vi "Get Device Info.vi"(8 "error in (no error)":errorcluster) -> (0 "error out":errorcluster, 2 "Success":bool, 3 "device info":T2 {"in_ver" format="%.2f"; "dr_ver" format="%.2f"; "fw_ver" format="%.2f"; "hw_ver" format="%.2f"})   [LabVIEW 2018, in "CAN FD.lvlib"]
uses:
  CAN FD.lvlib
  data_type/ZCAN_DEVICE_INFO.ctl
  bin/ControlCANFD.dll
panel:
  in  "ZCAN_DEVICE_INFO":T1
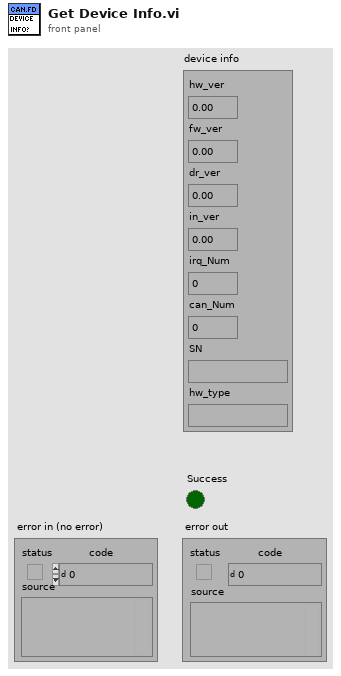
[diagram p1: front panel]
types:
  T1 = typedef "ZCAN_DEVICE_INFO.ctl" = cluster{"hw_Version":u16, "fw_Version":u16, "dr_Version":u16, "in_Version":u16, "irq_Num":u16, "can_Num":u8, "str_Serial_Num":cluster{"str_Serial_Num[0]":u8, "str_Serial_Num[1]":u8, "str_Serial_Num[2]":u8, "str_Serial_Num[3]":u8, "str_Serial_Num[4]":u8, "str_Serial_Num[5]":u8, "str_Serial_Num[6]":u8, "str_Serial_Num[7]":u8, "str_Serial_Num[8]":u8, "str_Serial_Num[9]":u8, "str_Serial_Num[10]":u8, "str_Serial_Num[11]":u8, "str_Serial_Num[12]":u8, "str_Serial_Num[13]":u8, "str_Serial_Num[14]":u8, "str_Serial_Num[15] ":u8, "str_Serial_Num[16] ":u8, "str_Serial_Num[17] ":u8, "str_Serial_Num[18] ":u8, "str_Serial_Num[19]":u8}, "str_hw_Type":cluster{"str_hw_Type[0]":u8, "str_hw_Type[1]":u8, "str_hw_Type[2]":u8, "str_hw_Type[3]":u8, "str_hw_Type[4]":u8, "str_hw_Type[5]":u8, "str_hw_Type[6]":u8, "str_hw_Type[7]":u8, "str_hw_Type[8]":u8, "str_hw_Type[9]":u8, "str_hw_Type[10]":u8, "str_hw_Type[11]":u8, "str_hw_Type[12]":u8, "str_hw_Type[13]":u8, "str_hw_Type[14]":u8, "str_hw_Type[15] ":u8, "str_hw_Type[16] ":u8, "str_hw_Type[17] ":u8, "str_hw_Type[18] ":u8, "str_hw_Type[19]":u8, "str_hw_Type[20]":u8, "str_hw_Type[21]":u8, "str_hw_Type[22]":u8, "str_hw_Type[23]":u8, "str_hw_Type[24]":u8, "str_hw_Type[25]":u8, "str_hw_Type[26]":u8, "str_hw_Type[27]":u8, "str_hw_Type[28]":u8, "str_hw_Type[29]":u8, "str_hw_Type[30]":u8, "str_hw_Type[31]":u8, "str_hw_Type[32]":u8, "str_hw_Type[33]":u8, "str_hw_Type[34]":u8, "str_hw_Type[35] ":u8, "str_hw_Type[36] ":u8, "str_hw_Type[37] ":u8, "str_hw_Type[38] ":u8, "str_hw_Type[39]":u8}, "reserved":cluster{"reserved[0]":u16, "reserved[1] ":u16, "reserved[2] ":u16, "reserved[3] ":u16}}
  T2 = cluster{"hw_ver":dbl, "fw_ver":dbl, "dr_ver":dbl, "in_ver":dbl, "irq_Num":u16, "can_Num":u8, "SN":string, "hw_type":string}
  T3 = cluster{"str_Serial_Num[0]":u8, "str_Serial_Num[1]":u8, "str_Serial_Num[2]":u8, "str_Serial_Num[3]":u8, "str_Serial_Num[4]":u8, "str_Serial_Num[5]":u8, "str_Serial_Num[6]":u8, "str_Serial_Num[7]":u8, "str_Serial_Num[8]":u8, "str_Serial_Num[9]":u8, "str_Serial_Num[10]":u8, "str_Serial_Num[11]":u8, "str_Serial_Num[12]":u8, "str_Serial_Num[13]":u8, "str_Serial_Num[14]":u8, "str_Serial_Num[15] ":u8, "str_Serial_Num[16] ":u8, "str_Serial_Num[17] ":u8, "str_Serial_Num[18] ":u8, "str_Serial_Num[19]":u8}
  T4 = cluster{"str_hw_Type[0]":u8, "str_hw_Type[1]":u8, "str_hw_Type[2]":u8, "str_hw_Type[3]":u8, "str_hw_Type[4]":u8, "str_hw_Type[5]":u8, "str_hw_Type[6]":u8, "str_hw_Type[7]":u8, "str_hw_Type[8]":u8, "str_hw_Type[9]":u8, "str_hw_Type[10]":u8, "str_hw_Type[11]":u8, "str_hw_Type[12]":u8, "str_hw_Type[13]":u8, "str_hw_Type[14]":u8, "str_hw_Type[15] ":u8, "str_hw_Type[16] ":u8, "str_hw_Type[17] ":u8, "str_hw_Type[18] ":u8, "str_hw_Type[19]":u8, "str_hw_Type[20]":u8, "str_hw_Type[21]":u8, "str_hw_Type[22]":u8, "str_hw_Type[23]":u8, "str_hw_Type[24]":u8, "str_hw_Type[25]":u8, "str_hw_Type[26]":u8, "str_hw_Type[27]":u8, "str_hw_Type[28]":u8, "str_hw_Type[29]":u8, "str_hw_Type[30]":u8, "str_hw_Type[31]":u8, "str_hw_Type[32]":u8, "str_hw_Type[33]":u8, "str_hw_Type[34]":u8, "str_hw_Type[35] ":u8, "str_hw_Type[36] ":u8, "str_hw_Type[37] ":u8, "str_hw_Type[38] ":u8, "str_hw_Type[39]":u8}
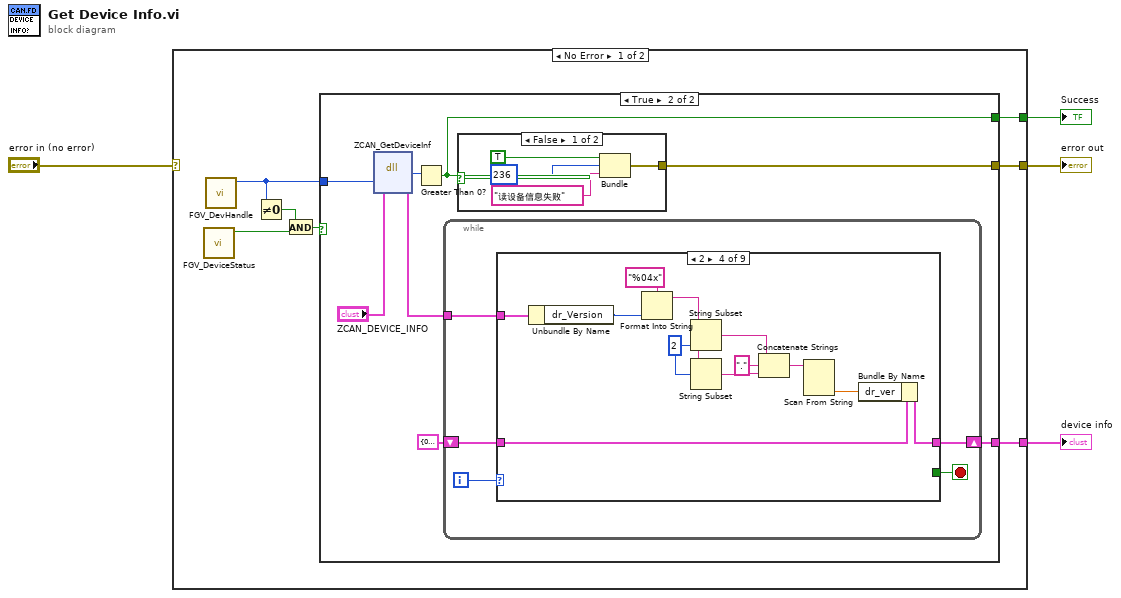
[diagram p0: block diagram]
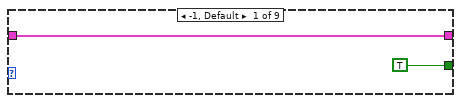
[diagram p3: hidden frame]
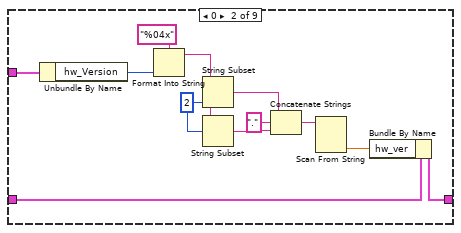
[diagram p4: hidden frame]
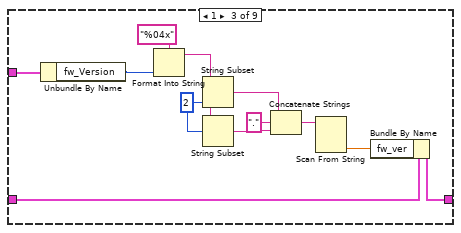
[diagram p5: hidden frame]
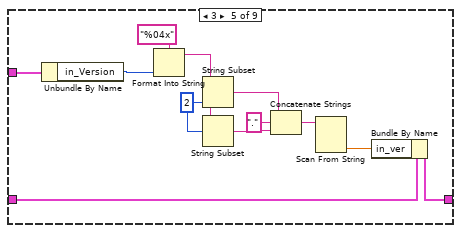
[diagram p6: hidden frame]
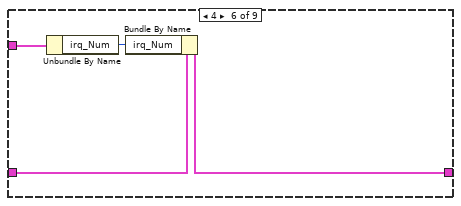
[diagram p7: hidden frame]
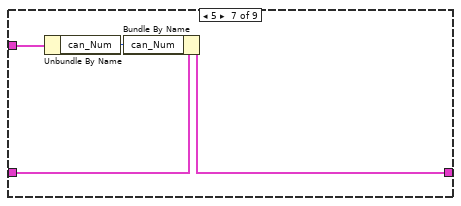
[diagram p8: hidden frame]
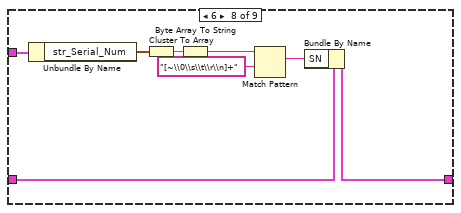
[diagram p9: hidden frame]
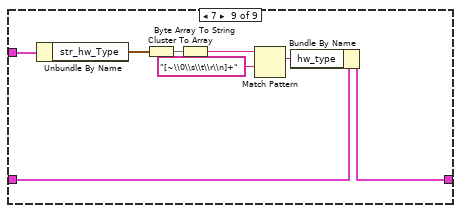
[diagram p10: hidden frame]
diagram:
  n1 = case shown="No Error" "error in (no error)" {
    selector: "error in (no error)" -> [_ w103]
    tunnel: [w8 w103] -> w4
    tunnel: [w7 _] -> w3
    tunnel: [w6 _] -> w2
    frame No Error {
      n2 = call "FGV_DeviceStatus.vi"() -> ("Open?"=w11:bool)  [unwired: 10 in, 1 out]
      n3 = call "FGV_DevHandle.vi"() -> ("handle out"=w9:u64)  [unwired: 9 in, 2 out]
      n4 = Not Equal To 0?(x=w9) -> (x != 0?=w10:bool)
      n5 = And(x=w10, y=w11) -> (x .and. y?=w5:bool)
      n6 = case shown="True" w5 {
        tunnel: w9 -> [_ w12]
        tunnel: [_ w17] -> w8
        tunnel: [_ w16] -> w7
        tunnel: [_ w14] -> w6
        frame False {
        }
        frame True {
          n7 = dll-call lib="C:/Users/ttc52/Desktop/DHC FD LV2018/LABIVIEW CANFD Tool_V1.2.4_20220724/bin/ControlCANFD.dll" fn="ZCAN_GetDeviceInf"("channel_handle"=w12, "pInfo"="ZCAN_DEVICE_INFO") -> ("return"=w19:u32, "pInfo"=w13:T1)  [unwired: 4 in, 2 out]
          n8 = Greater Than 0?(x=w19) -> (x > 0?=w16:bool)
          n9 = while {
            shift-right: [w23] -> w14
            shift-left: T2 {"hw_ver"=0.0, "fw_ver"=0.0, "dr_ver"=0.0, "in_ver"=0.0, "irq_Num"=0, "can_Num"=0, "SN"="", "hw_type"=""} ("device info") -> [w22]
            tunnel: w13 -> [w20]
            i -> [w24]
            stop <- w21 stop-if-true
            n10 = case shown="2" w24 {
              tunnel: [w26 w27 w39 w51 w63 w76 w80 w88 w96] -> w23
              tunnel: w22 -> [w26 w29 w41 w53 w65 w77 w81 w89 w97]
              tunnel: [TRUE _ _ _ _ _ _ _ _] -> w21
              tunnel: w20 -> [_ w38 w50 w62 w74 w78 w82 w90 w98]
              frame -1, Default {
              }
              frame 0 {
                w34 = 2 ("长度（剩余）")
                n11 = Unbundle By Name(w38) -> ("hw_Version"=w37:u16)
                n12 = Format Into String(format string="%04x" ("格式字符串"), w37) -> (resulting string=w35:string)  [unwired: 2 in, 1 out]
                n13 = String Subset(string=w35, length (rest)=w34) -> (substring=w32:string)  [unwired: 1 in]
                n14 = String Subset(string=w35, offset (0)=w34) -> (substring=w33:string)  [unwired: 1 in]
                n15 = Concatenate Strings(w32, "." ("字符串"), w33) -> (w30:string)
                n16 = Scan From String(input string=w30) -> (output 1=w28:dbl)  [unwired: 4 in, 3 out]
                n17 = Bundle By Name(cluster=w29, "hw_ver"=w28) -> (w27:T2)
              }
              frame 1 {
                w46 = 2 ("长度（剩余）")
                n18 = Unbundle By Name(w50) -> ("fw_Version"=w49:u16)
                n19 = Format Into String(format string="%04x" ("格式字符串"), w49) -> (resulting string=w47:string)  [unwired: 2 in, 1 out]
                n20 = String Subset(string=w47, length (rest)=w46) -> (substring=w44:string)  [unwired: 1 in]
                n21 = String Subset(string=w47, offset (0)=w46) -> (substring=w45:string)  [unwired: 1 in]
                n22 = Concatenate Strings(w44, "." ("字符串"), w45) -> (w42:string)
                n23 = Scan From String(input string=w42) -> (output 1=w40:dbl)  [unwired: 4 in, 3 out]
                n24 = Bundle By Name(cluster=w41, "fw_ver"=w40) -> (w39:T2)
              }
              frame 2 {
                w58 = 2 ("长度（剩余）")
                n25 = Unbundle By Name(w62) -> ("dr_Version"=w61:u16)
                n26 = Format Into String(format string="%04x" ("格式字符串"), w61) -> (resulting string=w59:string)  [unwired: 2 in, 1 out]
                n27 = String Subset(string=w59, length (rest)=w58) -> (substring=w56:string)  [unwired: 1 in]
                n28 = String Subset(string=w59, offset (0)=w58) -> (substring=w57:string)  [unwired: 1 in]
                n29 = Concatenate Strings(w56, "." ("字符串"), w57) -> (w54:string)
                n30 = Scan From String(input string=w54) -> (output 1=w52:dbl)  [unwired: 4 in, 3 out]
                n31 = Bundle By Name(cluster=w53, "dr_ver"=w52) -> (w51:T2)
              }
              frame 3 {
                w70 = 2 ("长度（剩余）")
                n32 = Unbundle By Name(w74) -> ("in_Version"=w73:u16)
                n33 = Format Into String(format string="%04x" ("格式字符串"), w73) -> (resulting string=w71:string)  [unwired: 2 in, 1 out]
                n34 = String Subset(string=w71, length (rest)=w70) -> (substring=w68:string)  [unwired: 1 in]
                n35 = String Subset(string=w71, offset (0)=w70) -> (substring=w69:string)  [unwired: 1 in]
                n36 = Concatenate Strings(w68, "." ("字符串"), w69) -> (w66:string)
                n37 = Scan From String(input string=w66) -> (output 1=w64:dbl)  [unwired: 4 in, 3 out]
                n38 = Bundle By Name(cluster=w65, "in_ver"=w64) -> (w63:T2)
              }
              frame 4 {
                n39 = Unbundle By Name(w78) -> ("irq_Num"=w75:u16)
                n40 = Bundle By Name(cluster=w77, "irq_Num"=w75) -> (w76:T2)
              }
              frame 5 {
                n41 = Unbundle By Name(w82) -> ("can_Num"=w79:u8)
                n42 = Bundle By Name(cluster=w81, "can_Num"=w79) -> (w80:T2)
              }
              frame 6 {
                n43 = Unbundle By Name(w90) -> ("str_Serial_Num"=w86:T3)
                n44 = Cluster To Array(cluster=w86) -> (array=w87:u8[])
                n45 = Byte Array To String(unsigned byte array=w87) -> (string=w85:string)
                n46 = Match Pattern(string=w85, regular expression="[~\\0\\s\\t\\r\\n]+" ("正则表达式")) -> (match substring=w83:string)  [unwired: 1 in, 3 out]
                n47 = Bundle By Name(cluster=w89, "SN"=w83) -> (w88:T2)
              }
              frame 7 {
                n48 = Unbundle By Name(w98) -> ("str_hw_Type"=w94:T4)
                n49 = Cluster To Array(cluster=w94) -> (array=w95:u8[])
                n50 = Byte Array To String(unsigned byte array=w95) -> (string=w93:string)
                n51 = Match Pattern(string=w93, regular expression="[~\\0\\s\\t\\r\\n]+" ("正则表达式")) -> (match substring=w91:string)  [unwired: 1 in, 3 out]
                n52 = Bundle By Name(cluster=w97, "hw_type"=w91) -> (w96:T2)
              }
            }
          }
          n53 = case shown="False" w16 {
            tunnel: [w99 _] -> w17
            frame False {
              n54 = Bundle("status"=TRUE, "code"=236, "消息"="读设备信息失败") -> (w99:cluster{"status":bool, "code":i32, "消息":string})  [unwired: 1 in]
            }
            frame True {
            }
          }
        }
      }
    }
    frame Error {
    }
  }
  "Success" <- w3
  "device info" <- w2
  "error out" <- w4
